vi "剖面停止.vi"(8 "error in (no error)":errorcluster) -> (0 "error out":errorcluster)   [LabVIEW 2016, in "elevator.lvlib"]
uses:
  elevator.lvlib
  DAM395CF/DAM395CF.lvlib
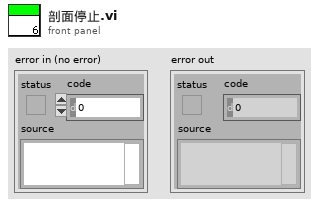
[diagram p1: front panel]
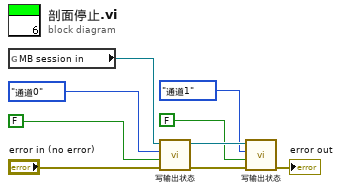
[diagram p0: block diagram]
diagram:
  n1 = global read "elevator 全局变量.vi" "MB session in"() -> (w1:refnum<class "MB_Master.lvclass">)
  n2 = call "写输出状态.vi"("error in (no error)"="error in (no error)", "value"=FALSE, "通道"=enum16{"通道0", "通道1", "通道2", "通道3"}."通道0", "MB session in"=w1) -> ("error out"=w5:errorcluster, "MB session out"=w7:refnum<class "MB_Master.lvclass">)  [unwired: 6 in]
  n3 = call "写输出状态.vi"("error in (no error)"=w5, "value"=FALSE, "通道"=enum16{"通道0", "通道1", "通道2", "通道3"}."通道1", "MB session in"=w7) -> ("error out"=→"error out":errorcluster)  [unwired: 6 in, 1 out]
